vi "Vision V5 2-15 (vascar would be V4) Windows.vi"(0 "Image in":T2(plugin-control), 5 "error in":errorcluster) -> (14 "Histogram (Histogram 1)":u32[][](array[numeric]), 15 "Shape Report (calibrated)":T1(array[cluster]) {"Score" format="%.2f"; "Centroid"."y" format="%.2f"; "Centroid"."x" format="%.2f"}, 16 "Number of Matches":i32, 19 "error out":errorcluster)   [LabVIEW 2019]
uses:
  <vilib>/Rock Robotics/Network Tables/NT Write Number.vi
  <vilib>/Rock Robotics/Network Tables/NT Read Number.vi
  <vilib>/Rock Robotics/Network Tables/NT Write String.vi
  <vilib>/Rock Robotics/Network Tables/NT Write Boolean.vi
  <vilib>/vision/NI_Vision_Development_Module.lvlib
panel:
  out "error out 2 (Path)":errorcluster
  in  "error in (no error) (Path)":errorcluster
  out "coerced(x)":sgl
  out "Image Out":T2(plugin-control)
  out "Histogram Graph":u32[][](graph)
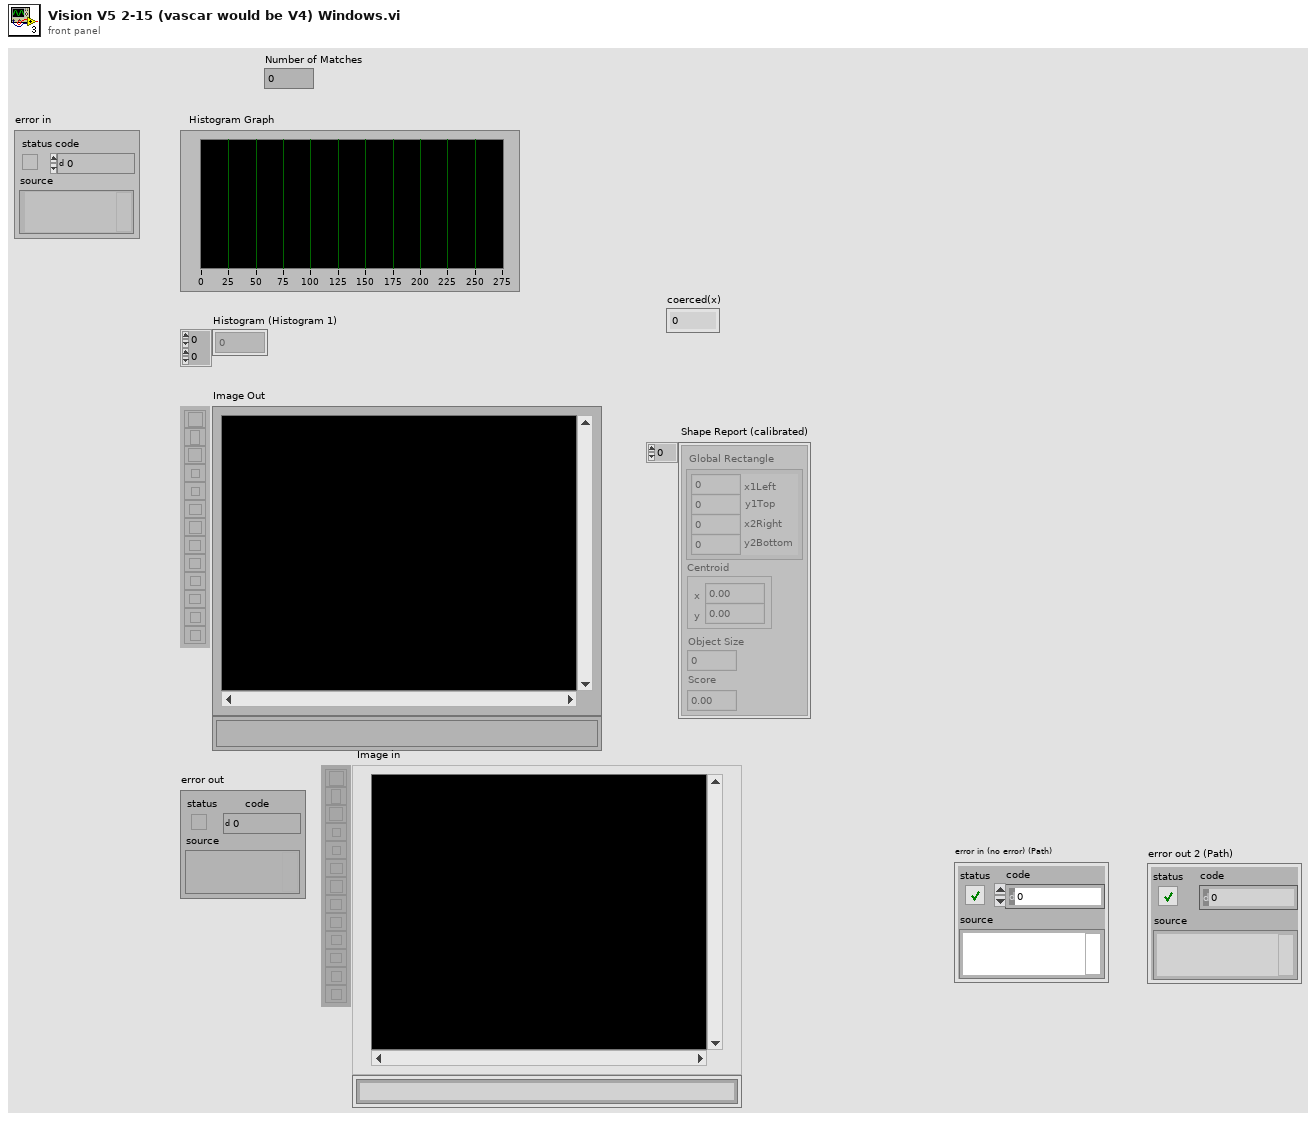
[diagram p1: front panel]
types:
  T1 = cluster{"Global Rectangle":cluster{"x1Left":i32, "y1Top":i32, "x2Right":i32, "y2Bottom":i32}, "Centroid":cluster{"x":sgl, "y":sgl}, "Object Size":u32, "Score":dbl}[]
  T2 = typedef "IMAQ Image.ctl" = refnum<image>
  T3 = cluster{"Measurement Parameter":i32, "Range Lower Value":dbl, "Range Upper Value":dbl, "Range":bool, "Measurement Type":bool}[]
  T4 = cluster{"Global Rectangle":i32[], "Contours":cluster{"ID":enum32{"External", "Internal"}, "Type":u32, "Coordinates":i32[]}[]}
  T5 = cluster{"Minimal Value":sgl, "Maximal Value":sgl, "Mean Value":sgl, "Standard  Variation":sgl, "Area (pixels)":i32}
  T6 = cluster{"histogram":u32[], "Minimal Value":sgl, "Maximal Value":sgl, "Starting Value":sgl, "Interval Width":sgl, "Mean Value":sgl, "Standard  Variation":sgl, "Area (pixels)":i32}
  T7 = typedef "Image Type" = u32
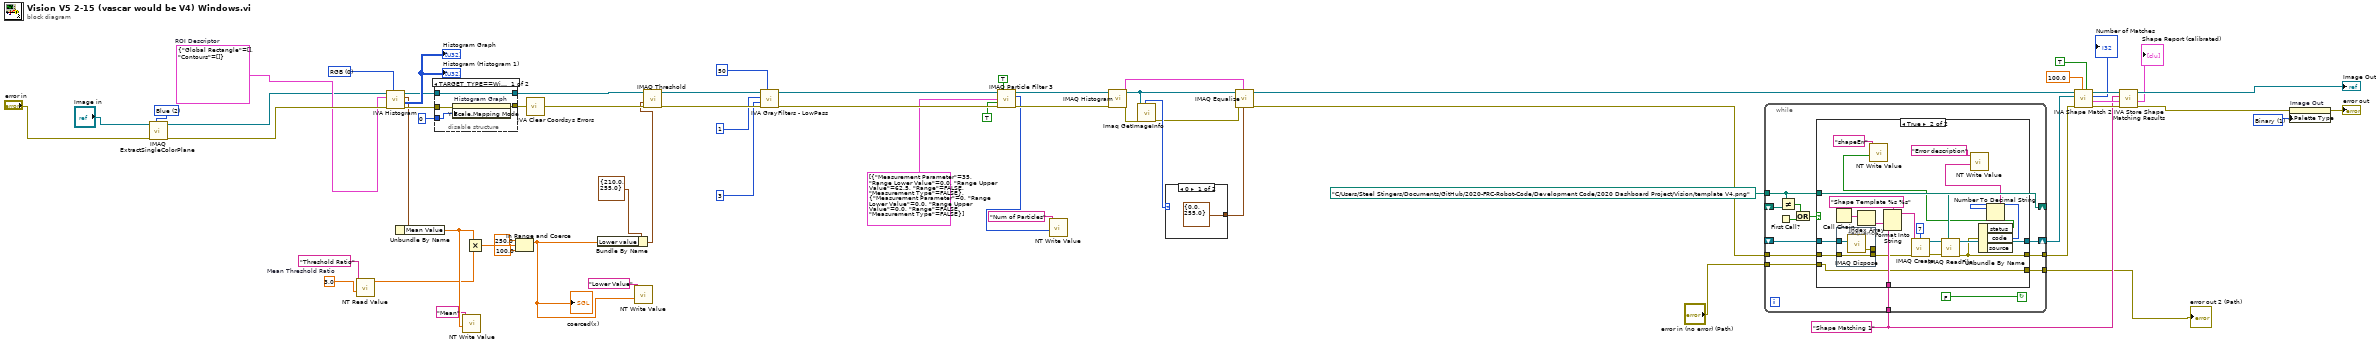
[diagram p0: block diagram]
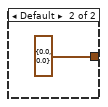
[diagram p3: hidden frame]
diagram:
  w4 = sgl 3.0  # Mean Threshold Ratio
  w23 = u32 1 items=["Grayscale", "Binary", "Gradient", "Rainbow", "Temperature", "User Defined", "Binary 16 Bit", "Gradient 16 Bit", "Rainbow 16 Bit", "Temperature 16 Bit", "User Defined 16 Bit"] ("Palette Type")
  w26 = "Shape Matching 1" ("Step Name")
  w62 = u16 0 items=["RGB", "HSL", "HSV", "HSI"] ("Color Mode")
  w60 = T4 {"Global Rectangle"=[], "Contours"=[]}  # ROI Descriptor
  w65 = 2 items=["Red", "Green", "Blue", "Hue", "Saturation", "Luminance", "Value", "Intensity"] ("Color Plane")
  n1 = call "IMAQ ExtractSingleColorPlane"("Color Plane"=w65, "error in (no error)"="error in", "Image Src"="Image in") -> ("error out"=w64:errorcluster, "Image Dst Out"=w1:T2)  [unwired: 1 in, 6 out]
  n2 = call-poly <vilib>:"NT Read Value.vi"("Default Value"=w4, "Name"="Threshold Ratio") -> ("Numeric"=w3:dbl)  [unwired: 8 in, 1 out]
  n3 = call <vilib>:"IVA Histogram.vi"("Color Mode"=w62, "error in (no error)"=w64, "ROI Descriptor"=w60, "Image In"=w1) -> ("error out"=w63:errorcluster, "Histograms"=→"Histogram Graph" →"Histogram (Histogram 1)":u32[][], "Statistics"=w22:T5, "Image Out"=w59:T2)  [unwired: 4 out]
  n4 = Unbundle By Name(w22) -> ("Mean Value"=w12:sgl)
  n5 = disable-structure "Conditional Disable Structure" shown="TARGET_TYPE==Windows" {
    disable-tunnel: w63 -> [w69 w70]
    disable-tunnel: [w68 w70] -> w57
    disable-tunnel: w59 -> [w67 w71]
    disable-tunnel: [w67 w71] -> w55
    disable-tunnel: u8 0 ("Y Scale.Mapping Mode") -> [w66 _]
    frame condition #0 (active) {
      n6 = property on="Histogram Graph" class="WFGraph (strict)"(error in=w69, "Y Scale.Mapping Mode"=w66) -> (error out=w68:errorcluster)  [unwired: 1 in, 1 out]
    }
    frame condition #1 {
    }
  }
  n7 = call-poly <vilib>:"NT Write Value.vi"("Numeric"=w12, "Name"="Mean") -> ()  [unwired: 9 in, 1 out]
  n8 = Multiply(x=w12, y=w3) -> (x*y=w20:dbl)
  n9 = In Range and Coerce(upper limit=sgl 250.0, x=w20, lower limit=sgl 100.0) -> (coerced(x)=w9:dbl)  [unwired: 1 out]
  "coerced(x)" <- w9
  n10 = call <vilib>:"IVA Clear Coordsys Errors.vi"("error in (no error)"=w57) -> ("error out"=w56:errorcluster)  [unwired: 10 in]
  n11 = Bundle By Name(cluster=cluster{"Lower value":sgl, "Upper value":sgl} {"Lower value"=210.0, "Upper value"=255.0} ("Range"), "Lower value"=w9) -> (w19:cluster{"Lower value":sgl, "Upper value":sgl})
  n12 = call-poly <vilib>:"NT Write Value.vi"("Numeric"=w9, "Name"="Lower Value") -> ()  [unwired: 9 in, 1 out]
  n13 = call "IMAQ Threshold"("error in (no error)"=w56, "Range"=w19, "Image Src"=w55) -> ("error out"=w54:errorcluster, "Image Dst Out"=w53:T2)  [unwired: 3 in, 4 out]
  n14 = call <vilib>:"IVA GrayFilters - LowPass.vi"("Tolerance"=50, "error in"=w54, "Filter size Y"=3, "Filter size X"=1, "Image In"=w53) -> ("error out"=w52:errorcluster, "Image Out"=w45:T2)  [unwired: 5 out]
  n15 = call "IMAQ Particle Filter 3"("Image Src"=w45, "Connectivity 4/8 (8)"=TRUE, "Selection Values"=T3 [{"Measurement Parameter"=35, "Range Lower Value"=0.0, "Range Upper Value"=62.5, "Range"=FALSE, "Measurement Type"=FALSE}, {"Measurement Parameter"=0, "Range Lower Value"=0.0, "Range Upper Value"=0.0, "Range"=FALSE, "Measurement Type"=FALSE}], "Keep/Remove Particles (F)"=TRUE ("Keep/Remove Particles"), "error in (no error)"=w52) -> ("Image Dst Out"=w40:T2, "Number of Particles"=w7:i32, "error out"=w46:errorcluster)  [unwired: 4 in, 4 out]
  n16 = call-poly <vilib>:"NT Write Value.vi"("Numeric"=w7, "Name"="Num of Particles") -> ()  [unwired: 9 in, 1 out]
  n17 = call "IMAQ Histogram"("error in (no error)"=w46, "Image"=w40) -> ("error out"=w39:errorcluster, "Histogram Report"=w42:T6)  [unwired: 3 in, 5 out]
  n18 = call "Imaq GetImageInfo"("error in (no error)"=w39, "Image"=w40) -> ("error out"=w38:errorcluster, "Image Type"=w41:T7)  [unwired: 8 out]
  n19 = case shown="0" w41 {
    tunnel: [cluster{"Minimum":sgl, "Maximum":sgl} {"Minimum"=0.0, "Maximum"=255.0} ("Range") cluster{"Minimum":sgl, "Maximum":sgl} {"Minimum"=0.0, "Maximum"=0.0} ("Range")] -> w37
    frame 0 {
    }
    frame Default {
    }
  }
  n20 = call "IMAQ Equalize"("Range"=w37, "Histogram Report"=w42, "error in (no error)"=w38, "Image Src"=w40) -> ("error out"=w43:errorcluster, "Image Dst Out"=w34:T2)  [unwired: 2 in, 4 out]
  n21 = while {
    shift-right: [w86] -> w27
    shift-left: _ -> [w85]
    tunnel: [w83] -> w28
    tunnel: w43 -> [w82]
    tunnel: path "C:/Users/Steel Stingers/Documents/GitHub/2020-FRC-Robot-Code/Development Code/2020 Dashboard Project/Vision/template V4.png" ("Template Path") -> [w80]
    tunnel: w26 -> [w81]
    shift-right: [w80] -> _
    shift-left: _ -> [w79]
    tunnel: [w75] -> w6
    tunnel: "error in (no error) (Path)" -> [w74]
    stop <- FALSE continue-if-true
    n22 = First Call?() -> (First Call?: T/F=w78:bool)
    n23 = Not Equal?(x=w80, y=w79) -> (x != y?=w77:bool)
    n24 = Or(x=w77, y=w78) -> (x .or. y?=w76:bool)
    n25 = case shown="True" w76 {
      tunnel: [w89 w106] -> w86
      tunnel: w85 -> [w89 w101]
      tunnel: [w88 w93] -> w83
      tunnel: w82 -> [w88 w100]
      tunnel: w80 -> [_ w94]
      tunnel: w81 -> [_ w102]
      tunnel: [w87 w98] -> w75
      tunnel: w74 -> [w87 w98]
      frame False {
      }
      frame True {
        n26 = Call Chain() -> (call chain=w104:string[])
        n27 = stacked-sequence {
          tunnel: w101 -> [w112]
          tunnel: w100 -> [w111]
          tunnel: [w111] -> w99
          tunnel: [w110] -> _
          frame #0 {
            n28 = call "IMAQ Dispose"("Image"=w112) -> ("error out"=w110:errorcluster)  [unwired: 2 in, 3 out]
          }
        }
        n29 = Index Array(array=w104) -> (element=w103:string)  [unwired: 1 in]
        n30 = Format Into String(format string="Shape Template %s %s" ("Image Name"), w103, w102) -> (resulting string=w109:string)  [unwired: 2 in, 1 out]
        n31 = call "IMAQ Create"("Border Size"=7, "Image Name"=w109, "error in (no error)"=w99) -> ("New Image"=w107:T2, "error out"=w95:errorcluster)  [unwired: 1 in, 1 out]
        n32 = call "IMAQ ReadFile"("File Path"=w94, "error in (no error)"=w95, "Image"=w107) -> ("error out"=w93:errorcluster, "Image Out"=w106:T2)  [unwired: 2 in, 5 out]
        n33 = Unbundle By Name(w93) -> ("status"=w92:bool, "code"=w91:i32)  [unwired: 1 out]
        n34 = call-poly <vilib>:"NT Write Value.vi"("Boolean"=w92, "Name"="shapeErr") -> ()  [unwired: 9 in, 1 out]
        n35 = Number To Decimal String(number=w91) -> (decimal integer string=w90:string)  [unwired: 1 in]
        n36 = call-poly <vilib>:"NT Write Value.vi"("String"=w90, "Name"="Error description") -> ()  [unwired: 9 in, 1 out]
      }
    }
  }
  "error out 2 (Path)" <- w6
  n37 = call <vilib>:"IVA Shape Match 2.vi"("Scale Invariance"=TRUE, "Minimal Score"=100.0, "error in (no error)"=w28, "Template"=w27, "Image Src"=w34) -> ("error out"=w33:errorcluster, "Shape Report"=w31:T1, "Number of Matches"=→"Number of Matches":i32, "Image Out"=w30:T2)  [unwired: 3 out]
  n38 = call <vilib>:"IVA Store Shape Matching Results.vi"("error in (no error)"=w33, "Shape Report"=w31, "Step Name"=w26, "Image in"=w30) -> ("error out"=w32:errorcluster, "Shape Report (calibrated)"=→"Shape Report (calibrated)":T1, "Image dup"=→"Image Out":T2)  [unwired: 5 out]
  n39 = property on="Image Out" class="ImageControl"(error in=w32, "Palette:Palette Type"=w23) -> (error out=→"error out":errorcluster)  [unwired: 1 in, 1 out]
